vi "Error Handling - Build Error.vi"(0 "Error Message":string, 1 "VI Path (calling VI path)":path, 2 "Error Code (-1300)":i32=-1300, 5 "error in (no error)":errorcluster, 6 "Create Error? (T)":bool=TRUE) -> (19 "error out":errorcluster)   [LabVIEW 2018]
doc: "This VI extends the functionality of the original build error VI. If no path is wired (default), then this VI will build the path to the calling VI. It will also create an error by default, so ideally, it should be used in a case structure only when an error is thrown, or the Create Error? input should be wired.\n\nThis VI is reentrant (shared clones)."
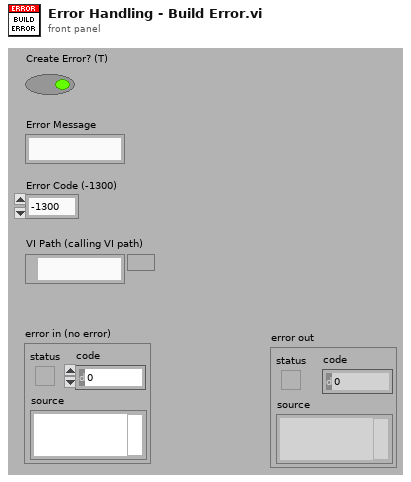
[diagram p1: front panel]
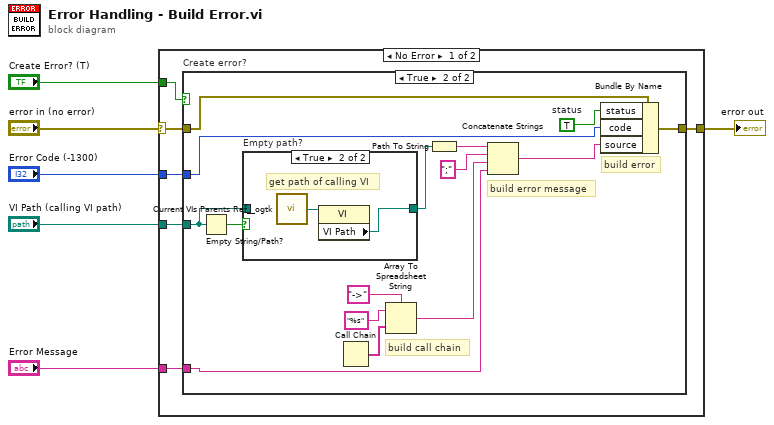
[diagram p0: block diagram]
diagram:
  n1 = case shown="No Error" "error in (no error)" {
    selector: "error in (no error)" -> [w10 w32]
    tunnel: [w8 w32] -> w6
    tunnel: "Error Message" -> [w12 _]
    tunnel: "Create Error? (T)" -> [w11 _]
    tunnel: "Error Code (-1300)" -> [w9 _]
    tunnel: "VI Path (calling VI path)" -> [w7 _]
    frame No Error {
      n2 = case "Create error?" shown="True" w11 {
        tunnel: w12 -> [_ w23]
        tunnel: w10 -> [w13 w18]
        tunnel: w9 -> [_ w21]
        tunnel: [w13 w19] -> w8
        tunnel: w7 -> [_ w14]
        frame False {
          # "do nothing"
        }
        frame True {
          w22 = TRUE  # status
          # "build error"
          # "build error message"
          # "build call chain"
          n3 = Empty String/Path?(string/path=w14) -> (empty?=w15:bool)
          n4 = case "Empty path?" shown="True" w15 {
            tunnel: [w29 w30] -> w17
            tunnel: w14 -> [w29 _]
            frame False {
              # "use wired path\nif not empty"
            }
            frame True {
              # "get path of calling VI"
              n5 = call <userlib>:"Current VIs Parents Ref__ogtk.vi"() -> ("Calling VI's Reference"=w31:refnum<vi>)  [unwired: 2 out]
              n6 = property class="VI"(reference=w31) -> ("VI Path"=w30:path)  [unwired: 1 in, 2 out]
            }
          }
          n7 = Call Chain() -> (call chain=w27:string[])
          n8 = Array To Spreadsheet String(delimiter (Tab)="->", array=w27, 3:"%s") -> (spreadsheet string=w28:string)
          n9 = Path To String(path=w17) -> (string=w16:string)
          n10 = Concatenate Strings(w16, ";", w28, w23) -> (w20:string)
          n11 = Bundle By Name(cluster=w18, "status"=w22, "code"=w21, "source"=w20) -> (w19:errorcluster)
        }
      }
    }
    frame Error {
    }
  }
  "error out" <- w6
